vi "REPLACE.vi"(7 "Actor in":refnum<class "Actor.lvclass">, 11 "Teardown State in":refnum<class "Teardown State.lvclass">) -> (2 "Destroy?":bool, 5 "Actor out":refnum<class "Actor.lvclass">)   [LabVIEW 2021, in "jettl.lvlib" / "Teardown State.lvclass"]
uses:
  Teardown State.lvclass
  Actor/Actor/Actor.lvclass
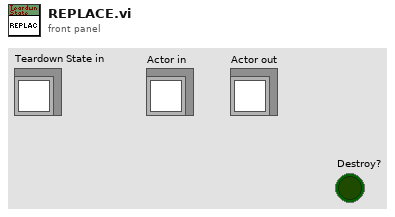
[diagram p1: front panel]
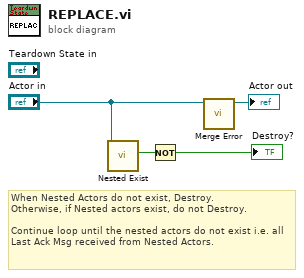
[diagram p0: block diagram]
diagram:
  # "When Nested Actors do not exist, Destroy.\nOtherwise, if Nested actors exist, do not Destroy.\n\nContinue loop until the nested actors do not exist i.e. all Last Ack Msg received from Nested Actors."
  n1 = call-dynamic "Nested Exist.vi"("Actor in"="Actor in") -> ("Nested Exist?"=w2:bool)  [unwired: 10 in]
  n2 = Not(x=w2) -> (.not. x?=→"Destroy?":bool)
  n3 = call-dynamic "Merge Error.vi"("Set Error in"="Actor in") -> ("Set Error out"=→"Actor out":refnum<class "Actor.lvclass">)  [unwired: 10 in]
